vi "Parse_Tag.vi"(0 "String":string) -> (2 "Item Type":T1, 3 "Item":string, 4 "Remaining String":string)   [LabVIEW 2011, in "Third Party VIs.lvlib" / "pcardinale.lvlib"]
uses:
  pcardinale.lvlib
  XML_Item_Type.ctl
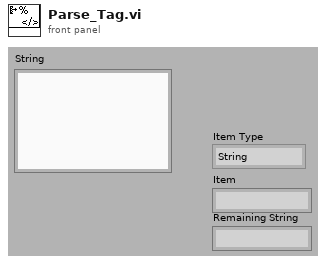
[diagram p1: front panel]
types:
  T1 = typedef "Third Party VIs.lvlib/pcardinale.lvlib/XML_Item_Type.ctl" = enum16{"String", "Start Tag", "Stop Tag", "Unified Tag"}
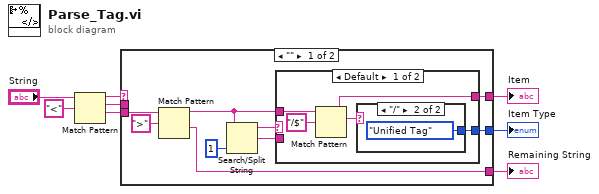
[diagram p0: block diagram]
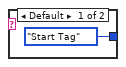
[diagram p2: hidden frame]
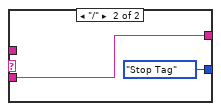
[diagram p3: hidden frame]
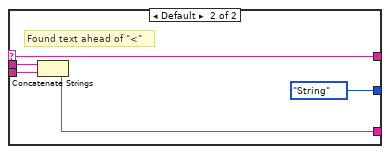
[diagram p4: hidden frame]
diagram:
  n1 = Match Pattern(string="String", regular expression="<" ("search string")) -> (before substring=w6:string, match substring=w5:string, after substring=w4:string)  [unwired: 1 in, 1 out]
  n2 = case shown="\"\"" w6 {
    selector: w6 -> [_ w29]
    tunnel: w5 -> [_ w31]
    tunnel: w4 -> [w17 w30]
    tunnel: [w14 w29] -> w3
    tunnel: [w15 w28] -> w2
    tunnel: [w9 XML_Item_Type."String" ("Item Type")] -> w1
    frame "" {
      n3 = Match Pattern(string=w17, regular expression=">") -> (before substring=w13:string, after substring=w15:string)  [unwired: 1 in, 2 out]
      n4 = Search/Split String(string=w13, offset (0)=1 ("length (rest)")) -> (substring before match=w11:string, match + rest of string=w10:string)  [unwired: 1 in, 1 out]
      n5 = case shown="Default" w11 {
        tunnel: w13 -> [w21 _]
        tunnel: [w19 w26] -> w14
        tunnel: w10 -> [_ w26]
        tunnel: [w22 XML_Item_Type."Stop Tag" ("Item Type")] -> w9
        frame Default {
          n6 = Match Pattern(string=w21, regular expression="/$") -> (before substring=w19:string, match substring=w18:string)  [unwired: 1 in, 2 out]
          n7 = case shown="\"/\"" w18 {
            tunnel: [XML_Item_Type."Start Tag" ("Item Type") XML_Item_Type."Unified Tag" ("Item Type")] -> w22
            frame Default {
            }
            frame "/" {
            }
          }
        }
        frame "/" {
        }
      }
    }
    frame Default {
      # "Found text ahead of \"<\""
      n8 = Concatenate Strings(w31, w30) -> (w28:string)
    }
  }
  "Item Type" <- w1
  "Item" <- w3
  "Remaining String" <- w2
